vi "Timothy CRD HF.vi"() -> (0 "error out":errorcluster)   [LabVIEW 2015]
uses:
  <vilib>/rvi/eio/nirviErrorMerge/nirviErrorMerge.xnode
  <vilib>/rvi/eio/common/nirviEmuClasses.ctl
  <vilib>/rvi/eio/common/nirviEmuTemplateMethod_errors.vi
  <vilib>/rvi/eio/nirviEIOMethodImplementation/nirviEIOMethodImplementation.xnode
  <vilib>/eio/EIOGrowableMethodNode/genericMethod/EIOGrowableMethodNode.xnode
  <vilib>/rvi/DataTransferAndStorage/Container/XNode/niFpgaContainer.xnode
  <vilib>/rvi/DataTransferAndStorage/Register/Emulation/niFpgaRegisterEmulation.vi
  <vilib>/eio/EIONode/EIONode.xnode
  <vilib>/rvi/interface/RandomDataEmulation/nirviRandomDataFpgaReadWriteTemplate.vi
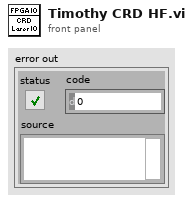
[diagram p1: front panel]
types:
  T1 = typedef "nirviEmuClasses.ctl" = enum16{"IO Read", "IO Write", "Method", "Property Read", "Property Write"}
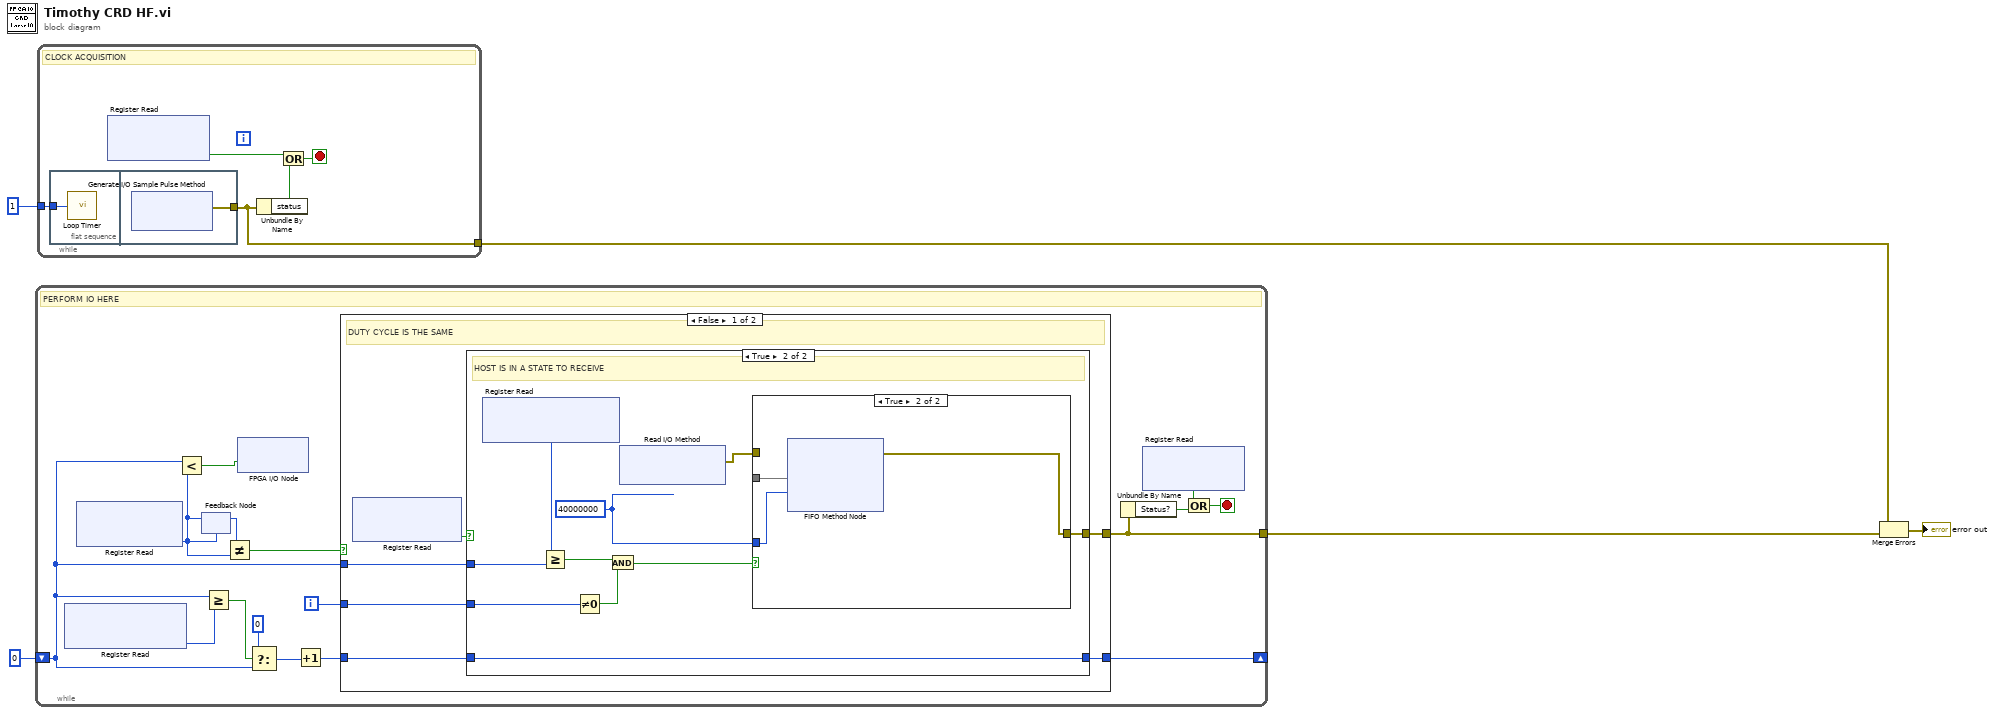
[diagram p0: block diagram]
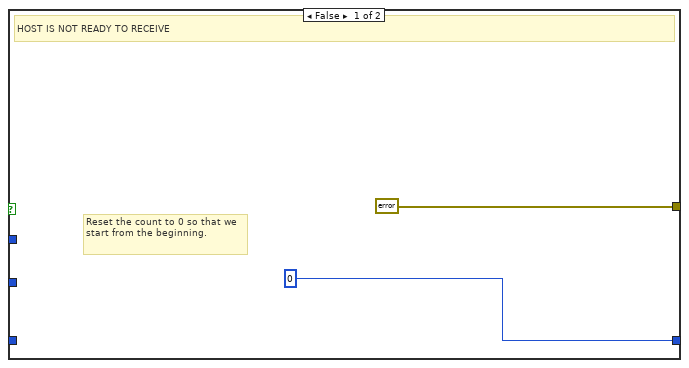
[diagram p2: hidden frame]
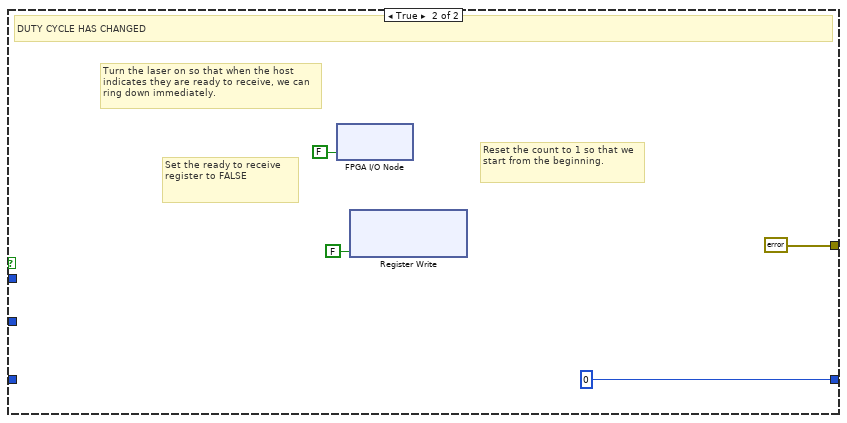
[diagram p4: hidden frame]
diagram:
  n1 = while {
    shift-right: [w11] -> _
    shift-left: u16 0 ("Number of Samples") -> [w15]
    tunnel: [w19] -> w1
    i -> [w6]
    stop <- w10 stop-if-true
    # "PERFORM IO HERE"
    n2 = xnode ("Register Read")() -> ("Data"=w16:u16)  [unwired: 1 in, 1 out]
    n3 = xnode ("Register Read")() -> ("Data"=w12:u16)  [unwired: 1 in, 1 out]
    n4 = Less?(x=w15, y=w12) -> (x < y?=w9:bool)
    n5 = feedback #1(w12) -> (w13:u16)
    n6 = feedback-in #1(w12) -> ()
    n7 = Greater Or Equal?(x=w15, y=w16) -> (x >= y?=w18:bool)
    n8 = Not Equal?(x=w13, y=w12) -> (x != y?=w14:bool)
    n9 = xnode "FPGA I/O Node"("Diode"=w9) -> ()  [unwired: 1 in, 1 out]
    n10 = Select(t=u16 0 ("Number of Samples"), s=w18, f=w15) -> (s? t:f=w8:u16)
    n11 = Increment(x=w8) -> (x+1=w7:u16)
    n12 = case shown="False" w14 {
      tunnel: [w27 errorcluster {"Status?"=FALSE, "Code"=0, "Source"=""} ("error out")] -> w19
      tunnel: w15 -> [w26 _]
      tunnel: w7 -> [w24 _]
      tunnel: [w23 u16 0 ("Number of Samples")] -> w11
      tunnel: w6 -> [w22 _]
      frame False {
        # "DUTY CYCLE IS THE SAME"
        n13 = xnode ("Register Read")() -> ("Data"=w25:bool)  [unwired: 1 in, 1 out]
        n14 = case shown="True" w25 {
          tunnel: [errorcluster {"Status?"=FALSE, "Code"=0, "Source"=""} ("error out") w35] -> w27
          tunnel: w26 -> [_ w33]
          tunnel: w24 -> [_ w40]
          tunnel: [u16 0 ("Number of Samples") w40] -> w23
          tunnel: w22 -> [_ w36]
          frame False {
            # "Reset the count to 0 so that we start from the beginning."
            # "HOST IS NOT READY TO RECEIVE"
          }
          frame True {
            w34 = 40000000 ("Timeout")
            # "HOST IS IN A STATE TO RECEIVE"
            n15 = xnode ("Register Read")() -> ("Data"=w32:u16)  [unwired: 1 in, 1 out]
            n16 = Greater Or Equal?(x=w32, y=w33) -> (x >= y?=w31:bool)
            n17 = Not Equal To 0?(x=w36) -> (x != 0?=w38:bool)
            n18 = And(x=w31, y=w38) -> (x .and. y?=w37:bool)
            n19 = xnode "Read I/O Method"(w34) -> ("error out"=w30:errorcluster)  [unwired: 1 in]
            n20 = case shown="True" w37 {
              tunnel: [_ w43] -> w39
              tunnel: [_ w41] -> w35
              tunnel: w34 -> [_ w42]
              tunnel: w30 -> [_ _]
              frame False {
              }
              frame True {
                n21 = xnode ("FIFO Method Node")("Element"=w43, "Timeout"=w42) -> ("error out"=w41:errorcluster)  [unwired: 2 in, 2 out]
              }
            }
          }
        }
      }
      frame True {
        # "Set the ready to receive register to FALSE"
        # "Reset the count to 1 so that we start from the beginning."
        # "Turn the laser on so that when the host indicates they are ready to receive, we can ring down immediately."
        # "DUTY CYCLE HAS CHANGED"
        n22 = xnode "FPGA I/O Node"("Diode"=FALSE) -> ()  [unwired: 1 in, 1 out]
        n23 = xnode ("Register Write")("Data"=FALSE) -> ()  [unwired: 1 in, 1 out]
      }
    }
    n24 = Unbundle By Name(w19) -> ("Status?"=w21:bool)
    n25 = xnode ("Register Read")() -> ("Data"=w17:bool)  [unwired: 1 in, 1 out]
    n26 = Compound Arithmetic op=OR(w17, w21) -> (w10:bool)
  }
  n27 = while {
    tunnel: u32 1 ("Sample Period (uSec)") -> [w123]
    tunnel: [w122] -> w5
    stop <- w119 stop-if-true
    # "CLOCK ACQUISITION"
    n28 = flat-sequence {
      tunnel: w123 -> [w124]
      tunnel: [w125] -> w122
      frame #0 {
        n29 = call "Loop Timer"("Count(uSec)"=w124) -> ()  [unwired: 1 out]
      }
      frame #1 {
        n30 = xnode "Generate I/O Sample Pulse Method"() -> ("error out"=w125:errorcluster)  [unwired: 1 in]
      }
    }
    n31 = xnode ("Register Read")() -> ("Data"=w121:bool)  [unwired: 1 in, 1 out]
    n32 = Unbundle By Name(w122) -> ("status"=w120:bool)
    n33 = Or(x=w121, y=w120) -> (x .or. y?=w119:bool)
  }
  n34 = Merge Errors(w5, w1) -> (→"error out":errorcluster)
